vi "Initialize System.vi"(4 "System Status":refnum<vi>, 6 "Error Queue":refnum<queue>, 8 "error in (no error)":errorcluster) -> (0 "error out":errorcluster)   [LabVIEW 2019]
uses:
  Variables/FGVs/Type Defs/FGV_Operations.ctl
  [meerstetter engineering TE Cooling]/TypeDefs/meTEC_Configuration.ctl
  Variables/Globals/Global_Initialized.vi
panel:
  # "--- Outputs ---"
  # "--- Inputs ---"
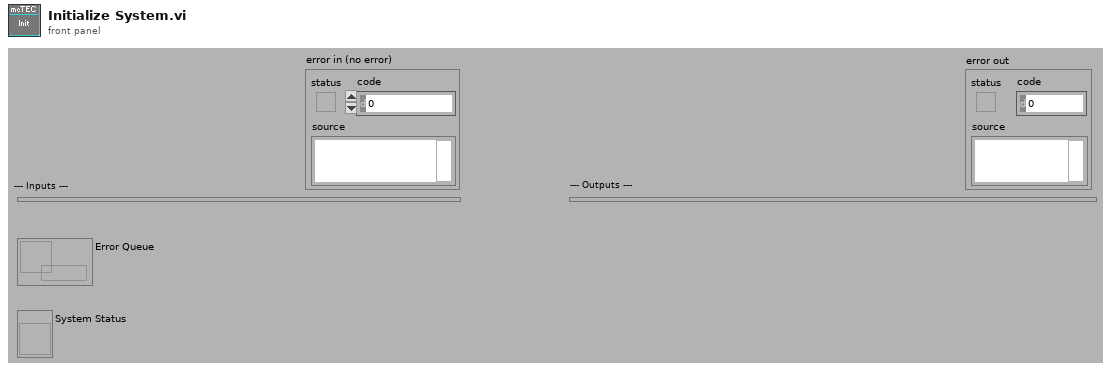
[diagram p1: front panel]
types:
  T1 = typedef "FGV_Operations.ctl" = enum16{"Read", "Write"}
  T2 = typedef "meTEC_Configuration.ctl" = cluster{"VISA resource name":refnum<visa-resource-name>, "Device Address":u16}
  T3 = typedef "FGV_TE Controller.ctl" = cluster{"SVs":cluster{"Unused":dbl}, "PVs":cluster{"FW & HW Versions":cluster{"Device Type [I32]":i32, "Device Type [String]":string, "Firmware Version [I32]":i32, "Firmware Version [String]":string, "Hardware Version [I32]":i32, "Hardware Version [String]":string, "Serial No.":i32}, "TEC Configuration":T2, "Object Target Temperature Source_CH1":u8, "Object Target Temperature Source_CH2":u8}, "Front Panel References":T4}
  T4 = typedef "FGV_Front Panel References.ctl" = cluster{"Main Loop Queue":refnum<queue>, "meTEC_Device Type":refnum<vi>, "meTEC_Serial No.":refnum<vi>, "meTEC_Hardware Version":refnum<vi>, "meTEC_Firmware Version":refnum<vi>, "meTEC_CH1_Object Target Temperature (ID 3000 / 50012) [°C]":refnum<vi>, "meTEC_CH1_Live Set Current (ID 50001) [A]":refnum<vi>, "meTEC_CH1_Live Set Voltage (ID 50002) [V]":refnum<vi>, "meTEC_CH1_Live Enable (ID 50000)":refnum<vi>, "meTEC_CH1_Input Selection (ID 2000)":refnum<vi>, "meTEC_CH1_Object Target Temp. Source Sel. (ID 50011)":refnum<vi>, "meTEC_CH2_Object Target Temperature (ID 3000 / 50012) [°C]":refnum<vi>, "meTEC_CH2_Live Set Current (ID 50001) [A]":refnum<vi>, "meTEC_CH2_Live Set Voltage (ID 50002) [V]":refnum<vi>, "meTEC_CH2_Live Enable (ID 50000)":refnum<vi>, "meTEC_CH2_Input Selection (ID 2000)":refnum<vi>, "meTEC_CH2_Object Target Temp. Source Sel. (ID 50011)":refnum<vi>, "meTEC_CH2_Object Temperature [°C]":refnum<vi>, "meTEC_CH2_Sink Temperature [°C]":refnum<vi>, "meTEC_CH2_Act. Output Current [A]":refnum<vi>, "meTEC_CH2_Act. Output Voltage [V]":refnum<vi>, "meTEC_CH2_Temperature Stability":refnum<vi>, "Monitor Chart_CH2":refnum<vi>, "meTEC_Initialize Device":refnum<vi>}
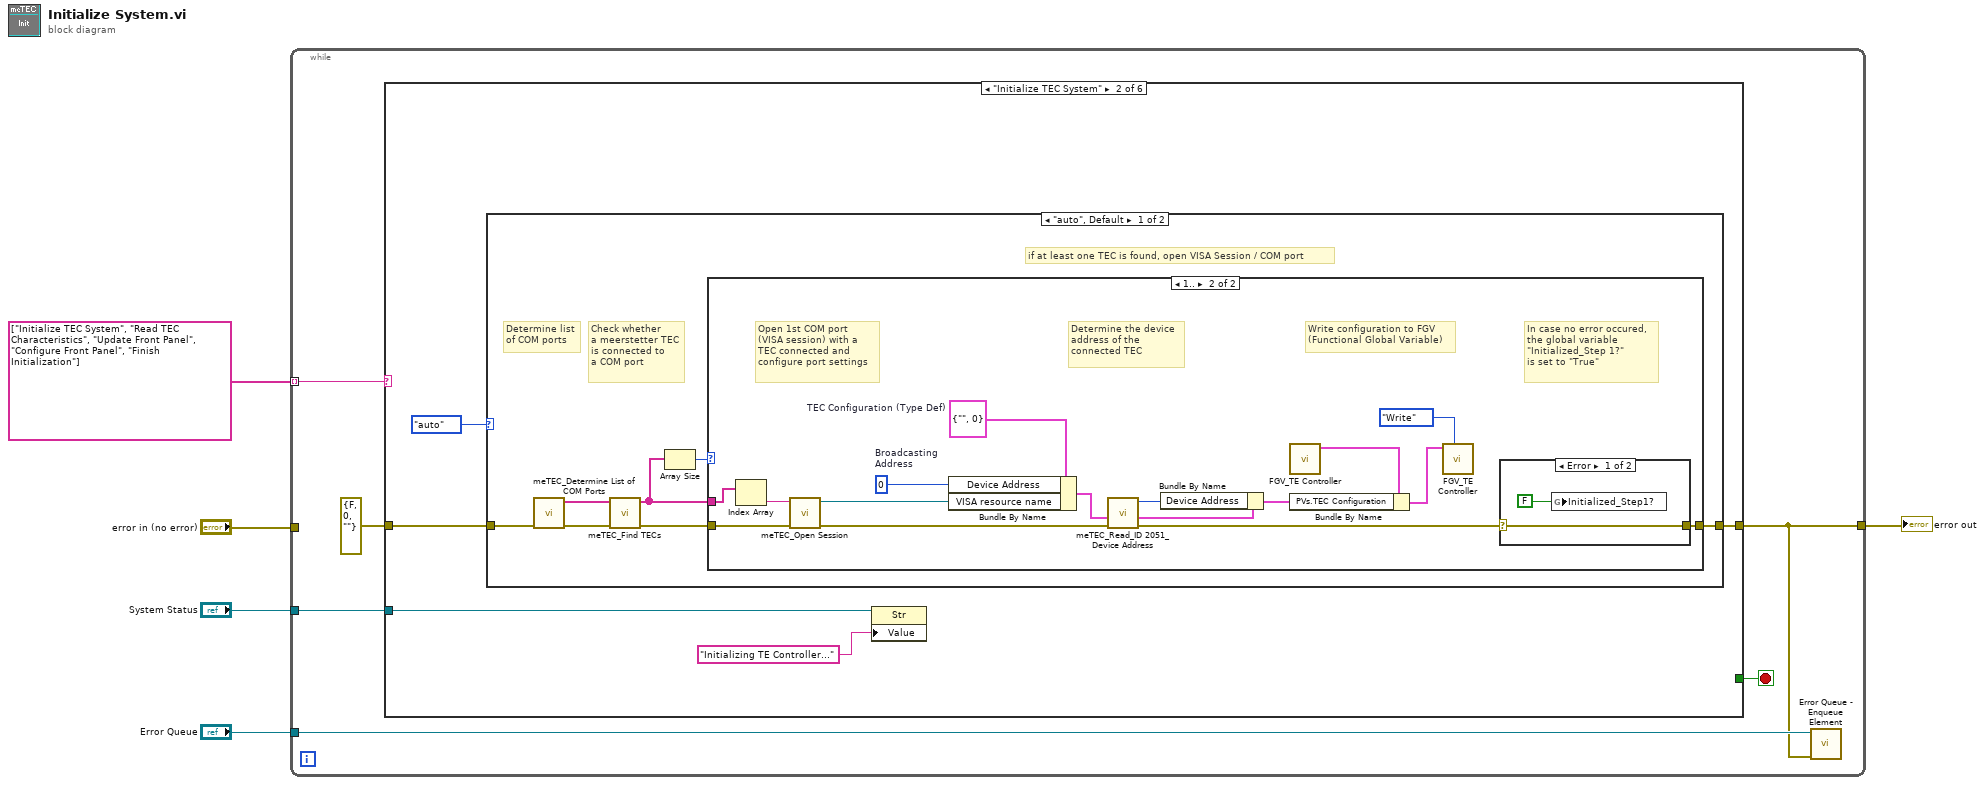
[diagram p0: block diagram]
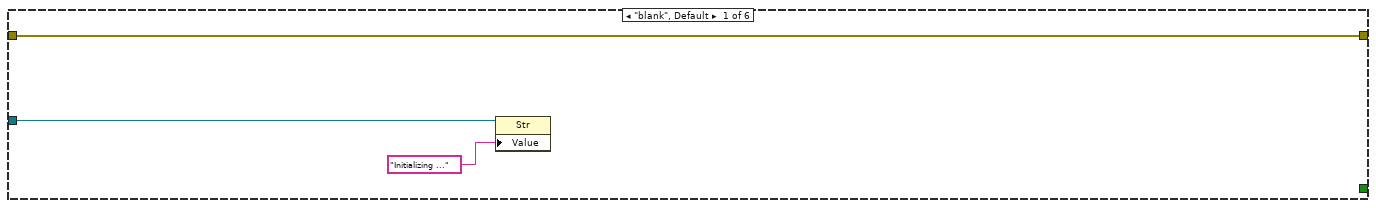
[diagram p2: hidden frame]
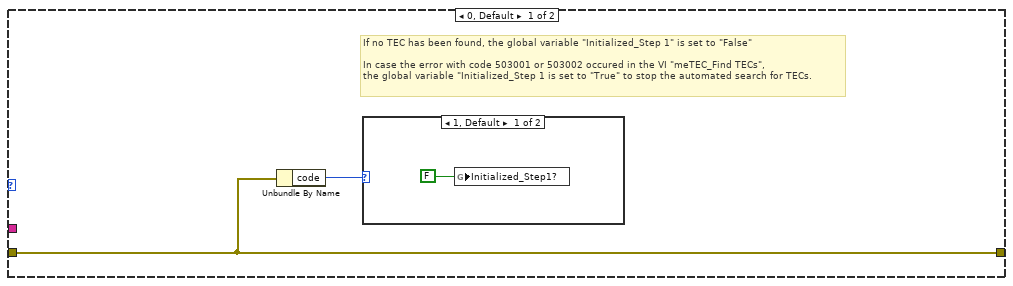
[diagram p3: hidden frame]
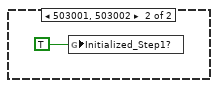
[diagram p4: hidden frame]
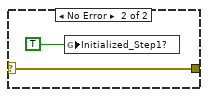
[diagram p5: hidden frame]
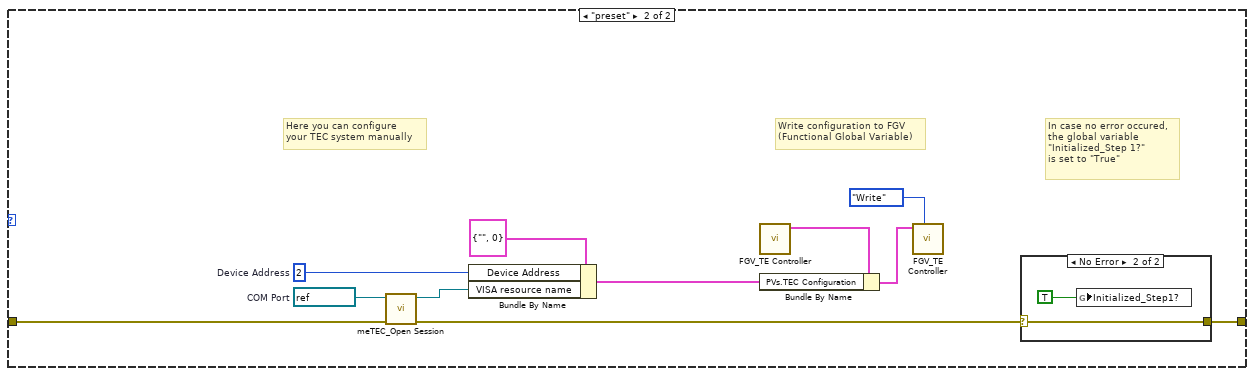
[diagram p6: hidden frame]
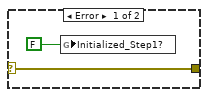
[diagram p7: hidden frame]
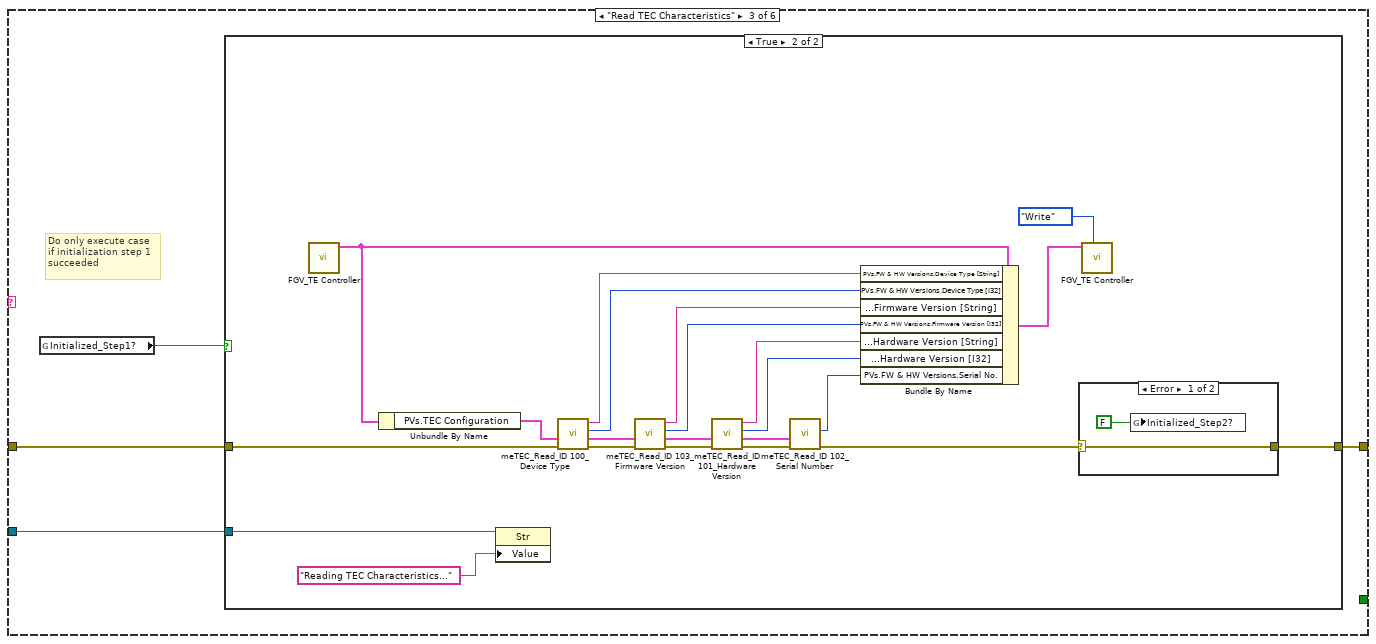
[diagram p8: hidden frame]
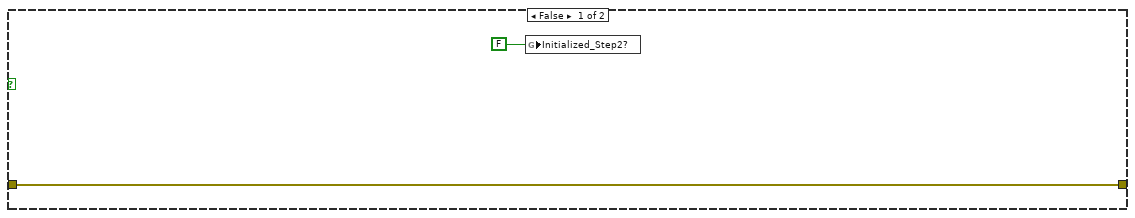
[diagram p9: hidden frame]
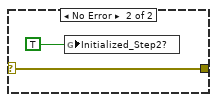
[diagram p10: hidden frame]
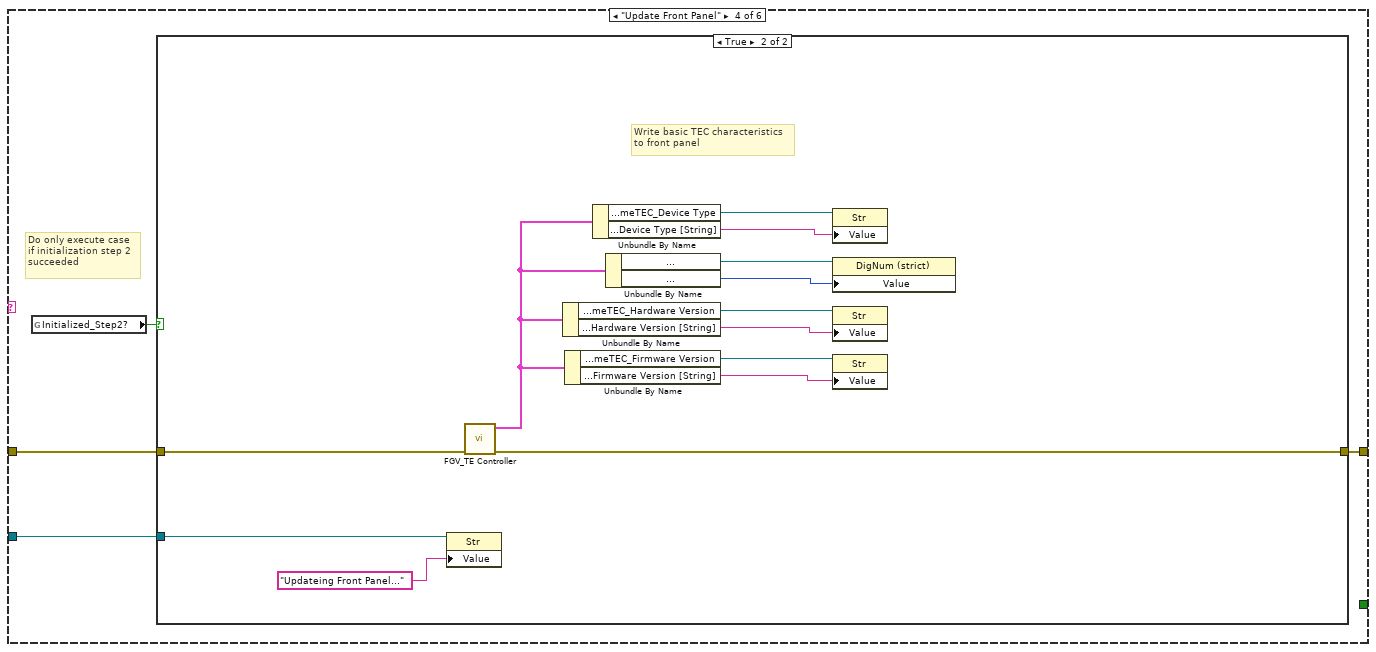
[diagram p11: hidden frame]
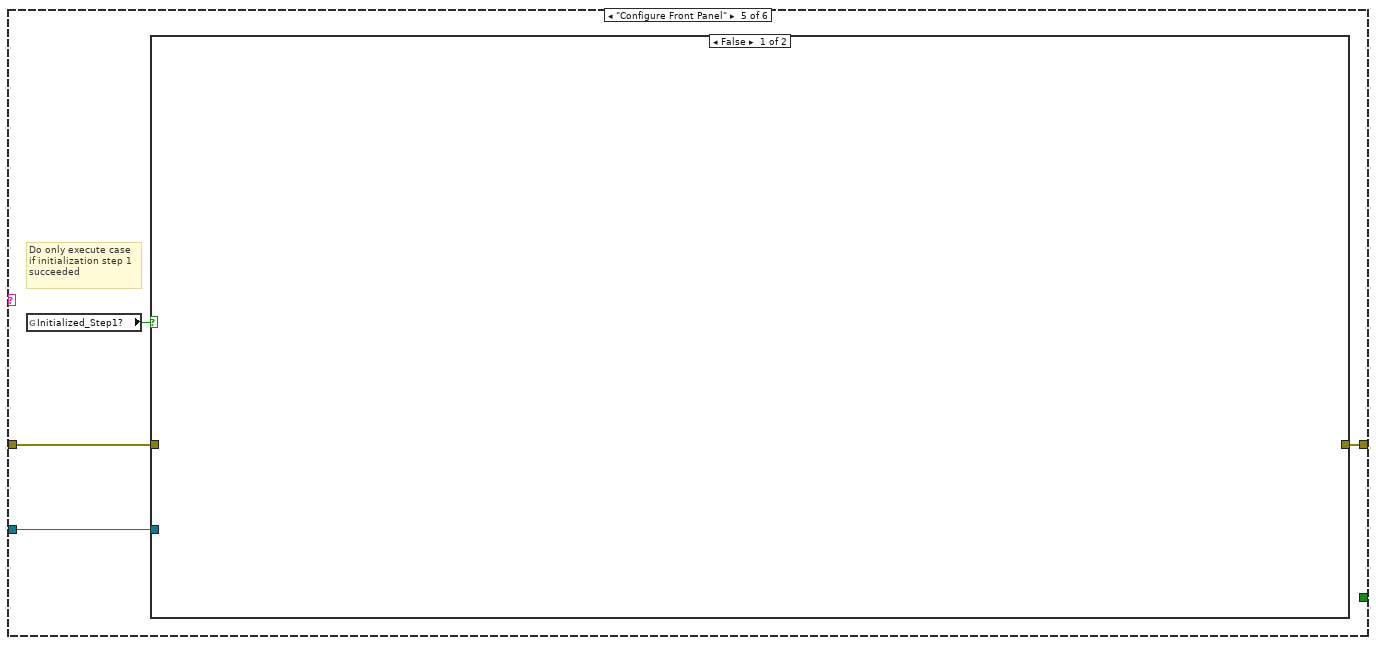
[diagram p13: hidden frame]
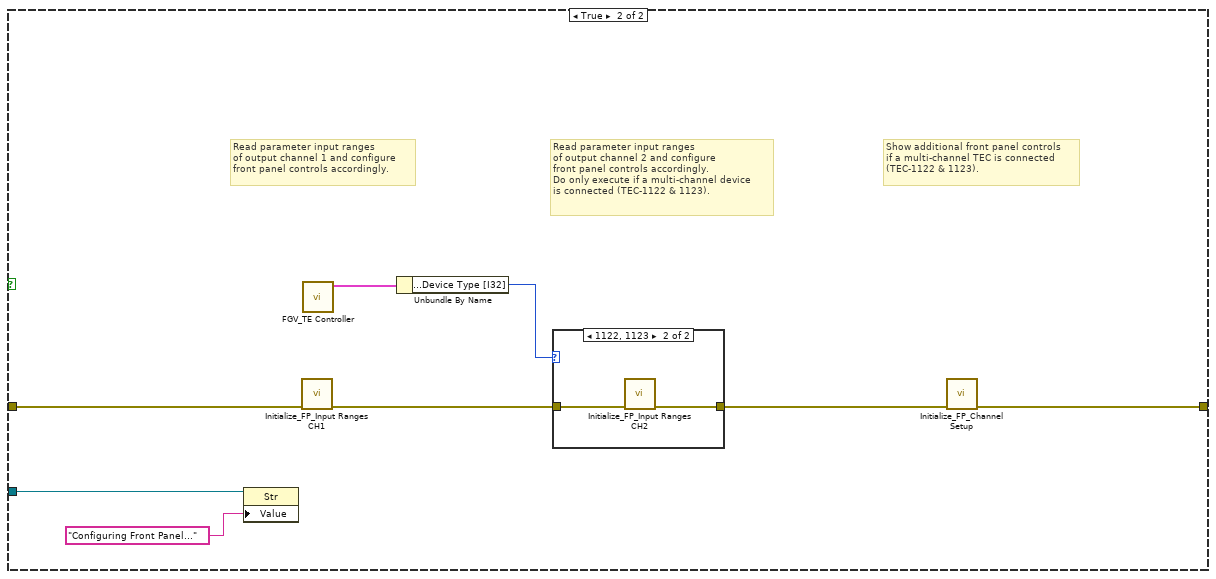
[diagram p14: hidden frame]
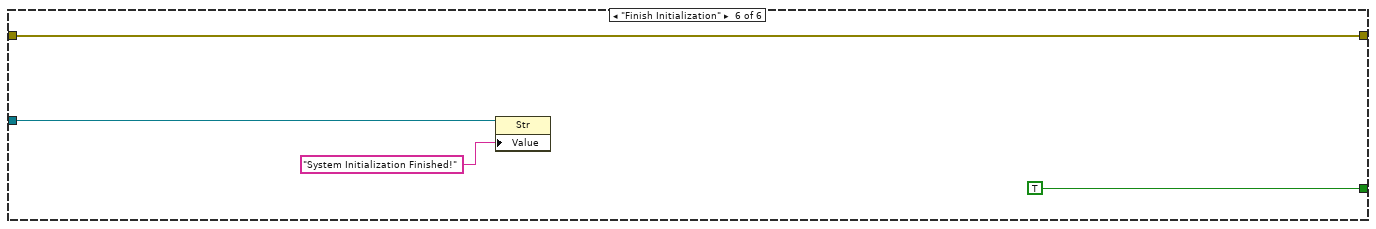
[diagram p16: hidden frame]
diagram:
  n1 = while {
    tunnel: "Error Queue" -> [w7]
    tunnel: string[] ["Initialize TEC System", "Read TEC Characteristics", "Update Front Panel", "Configure Front Panel", "Finish Initialization"] -> [w11] mode=indexing
    tunnel: "System Status" -> [w9]
    tunnel: "error in (no error)" -> [_]
    tunnel: [w6] -> w3
    stop <- w10 stop-if-true
    n2 = case shown="\"Initialize TEC System\"" w11 {
      tunnel: errorcluster {"status"=FALSE, "code"=0, "source"=""} ("error in (no error)") -> [w12 w17 w68 w98 w115 w131]
      tunnel: [w12 w15 w67 w100 w117 w131] -> w6
      tunnel: [_ _ _ _ _ TRUE ("status")] -> w10
      tunnel: w9 -> [w14 w19 w69 w101 w118 w132]
      frame "blank", Default {
        n3 = property class="Str"(reference=w14, "Value"="Initializing ...") -> ()  [unwired: 1 in, 2 out]
      }
      frame "Initialize TEC System" {
        n4 = case shown="\"auto\", Default" enum16{"auto", "preset"}."auto" {
          tunnel: w17 -> [w23 w57]
          tunnel: [w22 w52] -> w15
          frame "auto", Default {
            # "if at least one TEC is found, open VISA Session / COM port"
            # "Check whether\na meerstetter TEC\nis connected to\na COM port"
            # "Determine list\nof COM ports"
            n5 = call "meTEC_Determine List of COM Ports.vi"("error in (no error)"=w23) -> ("error out"=w26:errorcluster, "VISA Resources List (COM Ports)"=w25:string[])  [unwired: 9 in]
            n6 = call "meTEC_Find TECs.vi"("error in (no error)"=w26, "VISA Resources List (COM Ports)"=w25) -> ("error out"=w24:errorcluster, "VISA Resources List (meTEC(s))"=w21:string[])  [unwired: 8 in]
            n7 = Array Size(array=w21) -> (size(s)=w20:i32)
            n8 = case shown="1.." w20 {
              tunnel: w24 -> [w28 w46]
              tunnel: w21 -> [_ w45]
              tunnel: [w28 w32] -> w22
              frame 0, Default {
                # "If no TEC has been found, the global variable \"Initialized_Step 1\" is set to \"False\"\n\nIn case the error with code 503001 or 503002 occured in the VI \"meTEC_Find TECs\",\nthe global variable \"Initialized_Step 1 is set to \"True\" to stop the automated search for TECs."
                n9 = Unbundle By Name(w28) -> ("code"=w27:i32)
                n10 = case shown="1, Default" w27 {
                  frame 1, Default {
                    n11 = global write "Global_Initialized.vi" "Initialized_Step1?"(FALSE ("Initialized?")) -> ()
                  }
                  frame 503001, 503002 {
                    n12 = global write "Global_Initialized.vi" "Initialized_Step1?"(TRUE ("Initialized?")) -> ()
                  }
                }
              }
              frame 1.. {
                w44 = T2 {"VISA resource name"="", "Device Address"=0}  # TEC Configuration (Type Def)
                w43 = u16 0  # Broadcasting  Address
                # "In case no error occured,\nthe global variable\n\"Initialized_Step 1?\" \nis set to \"True\""
                # "Write configuration to FGV\n(Functional Global Variable)"
                # "Determine the device\naddress of the \nconnected TEC"
                # "Open 1st COM port\n(VISA session) with a\nTEC connected and\nconfigure port settings"
                n13 = Index Array(array=w45) -> (element=w33:string)  [unwired: 1 in]
                n14 = call "meTEC_Open Session.vi"("error in (no error)"=w46, "COM Port"=w33) -> ("error out"=w42:errorcluster, "VISA resource name_OUT"=w41:refnum<visa-resource-name>)  [unwired: 8 in]
                n15 = Bundle By Name(cluster=w44, "Device Address"=w43, "VISA resource name"=w41) -> (w40:T2)
                n16 = call "meTEC_Read_ID 2051_Device Address.vi"("error in (no error)"=w42, "TEC Configuration_IN"=w40) -> ("error out"=w31:errorcluster, "TEC Configuration_OUT"=w38:T2, "Device Address (ID 2051) [I32]"=w39:i32)  [unwired: 7 in]
                n17 = Bundle By Name(cluster=w38, "Device Address"=w39) -> (w34:T2)
                n18 = call "FGV_TE Controller.vi"() -> ("FGV_TEC_OUT"=w37:T3)  [unwired: 10 in, 1 out]
                n19 = Bundle By Name(cluster=w37, "PVs.TEC Configuration"=w34) -> (w36:T3)
                n20 = call "FGV_TE Controller.vi"("Operation (Read)"=FGV_Operations."Write", "FGV_TEC_IN"=w36) -> ()  [unwired: 8 in, 2 out]
                n21 = case shown="Error" w31 {
                  selector: w31 -> [w48 w50]
                  tunnel: [w48 w50] -> w32
                  frame Error {
                    n22 = global write "Global_Initialized.vi" "Initialized_Step1?"(FALSE ("Initialized?")) -> ()
                  }
                  frame No Error {
                    n23 = global write "Global_Initialized.vi" "Initialized_Step1?"(TRUE ("Initialized?")) -> ()
                  }
                }
              }
            }
          }
          frame "preset" {
            w59 = u16 2  # Device Address
            w61 = refnum<visa-resource-name> "COM4"  # COM Port
            # "In case no error occured,\nthe global variable\n\"Initialized_Step 1?\" \nis set to \"True\""
            # "Here you can configure\nyour TEC system manually"
            # "Write configuration to FGV\n(Functional Global Variable)"
            n24 = call "meTEC_Open Session.vi"("error in (no error)"=w57, "COM Port"=w61) -> ("error out"=w51:errorcluster, "VISA resource name_OUT"=w58:refnum<visa-resource-name>)  [unwired: 8 in]
            n25 = Bundle By Name(cluster=T2 {"VISA resource name"="", "Device Address"=0} ("TEC Configuration"), "Device Address"=w59, "VISA resource name"=w58) -> (w53:T2)
            n26 = call "FGV_TE Controller.vi"() -> ("FGV_TEC_OUT"=w56:T3)  [unwired: 10 in, 1 out]
            n27 = Bundle By Name(cluster=w56, "PVs.TEC Configuration"=w53) -> (w55:T3)
            n28 = call "FGV_TE Controller.vi"("Operation (Read)"=FGV_Operations."Write", "FGV_TEC_IN"=w55) -> ()  [unwired: 8 in, 2 out]
            n29 = case shown="No Error" w51 {
              selector: w51 -> [w63 w65]
              tunnel: [w63 w65] -> w52
              frame Error {
                n30 = global write "Global_Initialized.vi" "Initialized_Step1?"(FALSE ("Initialized?")) -> ()
              }
              frame No Error {
                n31 = global write "Global_Initialized.vi" "Initialized_Step1?"(TRUE ("Initialized?")) -> ()
              }
            }
          }
        }
        n32 = property class="Str"(reference=w19, "Value"="Initializing TE Controller...") -> ()  [unwired: 1 in, 2 out]
      }
      frame "Read TEC Characteristics" {
        # "Do only execute case\nif initialization step 1\nsucceeded"
        n33 = global read "Global_Initialized.vi" "Initialized_Step1?"() -> (w66:bool)
        n34 = case shown="True" w66 {
          tunnel: w69 -> [_ w93]
          tunnel: w68 -> [w71 w86]
          tunnel: [w71 w72] -> w67
          frame False {
            n35 = global write "Global_Initialized.vi" "Initialized_Step2?"(FALSE ("Initialized?")) -> ()
          }
          frame True {
            n36 = call "FGV_TE Controller.vi"() -> ("FGV_TEC_OUT"=w85:T3)  [unwired: 10 in, 1 out]
            n37 = Unbundle By Name(w85) -> ("PVs.TEC Configuration"=w84:T2)
            n38 = property class="Str"(reference=w93, "Value"="Reading TEC Characteristics...") -> ()  [unwired: 1 in, 2 out]
            n39 = call "meTEC_Read_ID 100_Device Type.vi"("error in (no error)"=w86, "TEC Configuration_IN"=w84) -> ("error out"=w89:errorcluster, "TEC Configuration_OUT"=w83:T2, "Device Type (ID 100) [I32]"=w74:i32, "Device Type (ID 100) [String]"=w75:string)  [unwired: 6 in]
            n40 = call "meTEC_Read_ID 103_Firmware Version.vi"("error in (no error)"=w89, "TEC Configuration_IN"=w83) -> ("error out"=w88:errorcluster, "TEC Configuration_OUT"=w82:T2, "Firmware Version (ID 103) [I32]"=w76:i32, "Firmware Version (ID 103) [String]"=w77:string)  [unwired: 6 in]
            n41 = call "meTEC_Read_ID 101_Hardware Version.vi"("error in (no error)"=w88, "TEC Configuration_IN"=w82) -> ("error out"=w87:errorcluster, "TEC Configuration_OUT"=w81:T2, "Hardware Version (ID 101) [I32]"=w78:i32, "Hardware Version (ID 101) [String]"=w79:string)  [unwired: 6 in]
            n42 = call "meTEC_Read_ID 102_Serial Number.vi"("error in (no error)"=w87, "TEC Configuration_IN"=w81) -> ("error out"=w73:errorcluster, "Serial No. (ID 102) [I32]"=w80:i32)  [unwired: 6 in, 2 out]
            n43 = Bundle By Name(cluster=w85, "PVs.FW & HW Versions.Device Type [String]"=w75, "PVs.FW & HW Versions.Device Type [I32]"=w74, "PVs.FW & HW Versions.Firmware Version [String]"=w77, "PVs.FW & HW Versions.Firmware Version [I32]"=w76, "PVs.FW & HW Versions.Hardware Version [String]"=w79, "PVs.FW & HW Versions.Hardware Version [I32]"=w78, "PVs.FW & HW Versions.Serial No."=w80) -> (w91:T3)
            n44 = case shown="Error" w73 {
              selector: w73 -> [w95 w97]
              tunnel: [w95 w97] -> w72
              frame Error {
                n45 = global write "Global_Initialized.vi" "Initialized_Step2?"(FALSE ("Initialized?")) -> ()
              }
              frame No Error {
                n46 = global write "Global_Initialized.vi" "Initialized_Step2?"(TRUE ("Initialized?")) -> ()
              }
            }
            n47 = call "FGV_TE Controller.vi"("Operation (Read)"=FGV_Operations."Write", "FGV_TEC_IN"=w91) -> ()  [unwired: 8 in, 2 out]
          }
        }
      }
      frame "Update Front Panel" {
        # "Do only execute case\nif initialization step 2\nsucceeded"
        n48 = global read "Global_Initialized.vi" "Initialized_Step2?"() -> (w99:bool)
        n49 = case shown="True" w99 {
          tunnel: w101 -> [_ w102]
          tunnel: [_ w114] -> w100
          tunnel: w98 -> [_ w104]
          frame False {
          }
          frame True {
            # "Write basic TEC characteristics\nto front panel"
            n50 = property class="Str"(reference=w102, "Value"="Updateing Front Panel...") -> ()  [unwired: 1 in, 2 out]
            n51 = call "FGV_TE Controller.vi"("error in (no error)"=w104) -> ("error out"=w114:errorcluster, "FGV_TEC_OUT"=w109:T3)  [unwired: 9 in]
            n52 = Unbundle By Name(w109) -> ("Front Panel References.meTEC_Hardware Version"=w108:refnum<vi>, "PVs.FW & HW Versions.Hardware Version [String]"=w107:string)
            n53 = Unbundle By Name(w109) -> ("Front Panel References.meTEC_Firmware Version"=w106:refnum<vi>, "PVs.FW & HW Versions.Firmware Version [String]"=w105:string)
            n54 = Unbundle By Name(w109) -> ("Front Panel References.meTEC_Device Type"=w113:refnum<vi>, "PVs.FW & HW Versions.Device Type [String]"=w112:string)
            n55 = Unbundle By Name(w109) -> ("Front Panel References.meTEC_Serial No."=w111:refnum<vi>, "PVs.FW & HW Versions.Serial No."=w110:i32)
            n56 = property on="Property Node" class="Str"(reference=w113, "Value"=w112) -> ()  [unwired: 1 in, 2 out]
            n57 = property on="Property Node" class="DigNum (strict)"(reference=w111, "Value"=w110) -> ()  [unwired: 1 in, 2 out]
            n58 = property on="Property Node" class="Str"(reference=w108, "Value"=w107) -> ()  [unwired: 1 in, 2 out]
            n59 = property on="Property Node" class="Str"(reference=w106, "Value"=w105) -> ()  [unwired: 1 in, 2 out]
          }
        }
      }
      frame "Configure Front Panel" {
        # "Do only execute case\nif initialization step 1\nsucceeded"
        n60 = global read "Global_Initialized.vi" "Initialized_Step1?"() -> (w116:bool)
        n61 = case shown="False" w116 {
          tunnel: w118 -> [_ w126]
          tunnel: [_ w123] -> w117
          tunnel: w115 -> [_ w124]
          frame False {
          }
          frame True {
            # "Read parameter input ranges\nof output channel 2 and configure\nfront panel controls accordingly.\nDo only execute if a multi-channel device\nis connected (TEC-1122 & 1123)."
            # "Read parameter input ranges\nof output channel 1 and configure\nfront panel controls accordingly."
            # "Show additional front panel controls\nif a multi-channel TEC is connected\n(TEC-1122 & 1123)."
            n62 = property class="Str"(reference=w126, "Value"="Configuring Front Panel...") -> ()  [unwired: 1 in, 2 out]
            n63 = call "Initialize_FP_Input Ranges CH1.vi"("error in (no error)"=w124) -> ("error out"=w122:errorcluster)  [unwired: 10 in]
            n64 = call "FGV_TE Controller.vi"() -> ("FGV_TEC_OUT"=w120:T3)  [unwired: 10 in, 1 out]
            n65 = Unbundle By Name(w120) -> ("PVs.FW & HW Versions.Device Type [I32]"=w119:i32)
            n66 = case shown="1122, 1123" w119 {
              tunnel: w122 -> [w127 w129]
              tunnel: [w127 w128] -> w121
              frame 1089..1091, Default {
              }
              frame 1122, 1123 {
                n67 = call "Initialize_FP_Input Ranges CH2.vi"("error in (no error)"=w129) -> ("error out"=w128:errorcluster)  [unwired: 10 in]
              }
            }
            n68 = call "Initialize_FP_Channel Setup.vi"("error in (no error)"=w121) -> ("error out"=w123:errorcluster)  [unwired: 10 in]
          }
        }
      }
      frame "Finish Initialization" {
        n69 = property class="Str"(reference=w132, "Value"="System Initialization Finished!") -> ()  [unwired: 1 in, 2 out]
      }
    }
    n70 = call "Error Queue - Enqueue Element.vi"("error in (no error)"=w6, "Error Queue IN"=w7) -> ()  [unwired: 9 in, 1 out]
  }
  "error out" <- w3
